vi "FGV Drift Daten.vi"(0 "SpanRegister":refnum<vi>, 1 "0-Gas Wert?":bool, 5 "Testnr.":i32, 7 "Drift Konfig Daten":T10={"Bearbeiter:"="", "Pfad:"=path "D:/IAG_Data/Log", "Textname:"="", "CG Aufschaltzeit:"=120.0, "N2 Aufschaltzeit:"=120.0} {"N2 Aufschaltzeit:" min=10.0; "CG Aufschaltzeit:" min=10.0}, 9 "Spangaseinstellungen":T2[](array[typedef]) {"Komponenten"."Komponente 5"."Komponente:" items=["NO (350,3000) LP 191C", "NO2 (150) LP 191C (1of2)", "NO2 (2000) LP 191C (2of2)", "N2O (300) LP 191C (1of2)", "NH3 (300) LP 191C (1of2)", "NH3 (900,3000) LP 191C (2of2)", "HNCO (400) 191C", "H2O% (30) LP 191C", "Formaldehyde (70,500) LP 191C", "CO2 low% (4) LP 191C (2of2)", "CO2% (20) LP 191C (1of2)", "CO (700) LP 191C (1of3)", "CO% (1) LP 191C (2of3)", "Propylene (1000) LP 191C", "Aromatic HC C7 (500) LP 191C", "Ethylene (1000) LP 191C", "CH4 (250) LP 191C (1of2)", "CH4 (5000) LP 191C (2of2)", "Ethane (1000) LP 191C", "Acetylene (1000) LP 191C", "HNO2 (20) 191C", "MeOH (1000) 191C", "CO% (10) LP 191C (3of3)", "Formic Acid (100) 191C", "SO2 (500) LP 191C", "Acetaldehyde (1000) LP 191C", "COS (100) LP 191C", "1,3 butadiene (100) LP 191C", "Oil as Octane (200) LP 191C", "N2O (1000) LP 191C (2of2)", "Propane (200) LP 191C", "NO2 autorange (2000)", "CO autorange (100000)", "CH4 autorange (5000)", "NH3 autorange (3000)", "Temp. Gascell", "Pressure Gascell", "sBeam@2500"]; "Komponenten"."Komponente 5"."Konzentration IST" format="%#.4f"; "Komponenten"."Komponente 5"."Genauigkeit" format="%#.1f"; "Komponenten"."Komponente 4"."Komponente:" items=["NO (350,3000) LP 191C", "NO2 (150) LP 191C (1of2)", "NO2 (2000) LP 191C (2of2)", "N2O (300) LP 191C (1of2)", "NH3 (300) LP 191C (1of2)", "NH3 (900,3000) LP 191C (2of2)", "HNCO (400) 191C", "H2O% (30) LP 191C", "Formaldehyde (70,500) LP 191C", "CO2 low% (4) LP 191C (2of2)", "CO2% (20) LP 191C (1of2)", "CO (700) LP 191C (1of3)", "CO% (1) LP 191C (2of3)", "Propylene (1000) LP 191C", "Aromatic HC C7 (500) LP 191C", "Ethylene (1000) LP 191C", "CH4 (250) LP 191C (1of2)", "CH4 (5000) LP 191C (2of2)", "Ethane (1000) LP 191C", "Acetylene (1000) LP 191C", "HNO2 (20) 191C", "MeOH (1000) 191C", "CO% (10) LP 191C (3of3)", "Formic Acid (100) 191C", "SO2 (500) LP 191C", "Acetaldehyde (1000) LP 191C", "COS (100) LP 191C", "1,3 butadiene (100) LP 191C", "Oil as Octane (200) LP 191C", "N2O (1000) LP 191C (2of2)", "Propane (200) LP 191C", "NO2 autorange (2000)", "CO autorange (100000)", "CH4 autorange (5000)", "NH3 autorange (3000)", "Temp. Gascell", "Pressure Gascell", "sBeam@2500"]; "Komponenten"."Komponente 4"."Konzentration IST" format="%#.4f"; "Komponenten"."Komponente 4"."Genauigkeit" format="%#.1f"; "Komponenten"."Komponente 3"."Komponente:" items=["NO (350,3000) LP 191C", "NO2 (150) LP 191C (1of2)", "NO2 (2000) LP 191C (2of2)", "N2O (300) LP 191C (1of2)", "NH3 (300) LP 191C (1of2)", "NH3 (900,3000) LP 191C (2of2)", "HNCO (400) 191C", "H2O% (30) LP 191C", "Formaldehyde (70,500) LP 191C", "CO2 low% (4) LP 191C (2of2)", "CO2% (20) LP 191C (1of2)", "CO (700) LP 191C (1of3)", "CO% (1) LP 191C (2of3)", "Propylene (1000) LP 191C", "Aromatic HC C7 (500) LP 191C", "Ethylene (1000) LP 191C", "CH4 (250) LP 191C (1of2)", "CH4 (5000) LP 191C (2of2)", "Ethane (1000) LP 191C", "Acetylene (1000) LP 191C", "HNO2 (20) 191C", "MeOH (1000) 191C", "CO% (10) LP 191C (3of3)", "Formic Acid (100) 191C", "SO2 (500) LP 191C", "Acetaldehyde (1000) LP 191C", "COS (100) LP 191C", "1,3 butadiene (100) LP 191C", "Oil as Octane (200) LP 191C", "N2O (1000) LP 191C (2of2)", "Propane (200) LP 191C", "NO2 autorange (2000)", "CO autorange (100000)", "CH4 autorange (5000)", "NH3 autorange (3000)", "Temp. Gascell", "Pressure Gascell", "sBeam@2500"]; "Komponenten"."Komponente 3"."Konzentration IST" format="%#.4f"; "Komponenten"."Komponente 3"."Genauigkeit" format="%#.1f"; "Komponenten"."Komponente 2"."Komponente:" items=["NO (350,3000) LP 191C", "NO2 (150) LP 191C (1of2)", "NO2 (2000) LP 191C (2of2)", "N2O (300) LP 191C (1of2)", "NH3 (300) LP 191C (1of2)", "NH3 (900,3000) LP 191C (2of2)", "HNCO (400) 191C", "H2O% (30) LP 191C", "Formaldehyde (70,500) LP 191C", "CO2 low% (4) LP 191C (2of2)", "CO2% (20) LP 191C (1of2)", "CO (700) LP 191C (1of3)", "CO% (1) LP 191C (2of3)", "Propylene (1000) LP 191C", "Aromatic HC C7 (500) LP 191C", "Ethylene (1000) LP 191C", "CH4 (250) LP 191C (1of2)", "CH4 (5000) LP 191C (2of2)", "Ethane (1000) LP 191C", "Acetylene (1000) LP 191C", "HNO2 (20) 191C", "MeOH (1000) 191C", "CO% (10) LP 191C (3of3)", "Formic Acid (100) 191C", "SO2 (500) LP 191C", "Acetaldehyde (1000) LP 191C", "COS (100) LP 191C", "1,3 butadiene (100) LP 191C", "Oil as Octane (200) LP 191C", "N2O (1000) LP 191C (2of2)", "Propane (200) LP 191C", "NO2 autorange (2000)", "CO autorange (100000)", "CH4 autorange (5000)", "NH3 autorange (3000)", "Temp. Gascell", "Pressure Gascell", "sBeam@2500"]; "Komponenten"."Komponente 2"."Konzentration IST" format="%#.4f"; "Komponenten"."Komponente 2"."Genauigkeit" format="%#.1f"; "Komponenten"."Komponente 1"."Komponente:" items=["NO (350,3000) LP 191C", "NO2 (150) LP 191C (1of2)", "NO2 (2000) LP 191C (2of2)", "N2O (300) LP 191C (1of2)", "NH3 (300) LP 191C (1of2)", "NH3 (900,3000) LP 191C (2of2)", "HNCO (400) 191C", "H2O% (30) LP 191C", "Formaldehyde (70,500) LP 191C", "CO2 low% (4) LP 191C (2of2)", "CO2% (20) LP 191C (1of2)", "CO (700) LP 191C (1of3)", "CO% (1) LP 191C (2of3)", "Propylene (1000) LP 191C", "Aromatic HC C7 (500) LP 191C", "Ethylene (1000) LP 191C", "CH4 (250) LP 191C (1of2)", "CH4 (5000) LP 191C (2of2)", "Ethane (1000) LP 191C", "Acetylene (1000) LP 191C", "HNO2 (20) 191C", "MeOH (1000) 191C", "CO% (10) LP 191C (3of3)", "Formic Acid (100) 191C", "SO2 (500) LP 191C", "Acetaldehyde (1000) LP 191C", "COS (100) LP 191C", "1,3 butadiene (100) LP 191C", "Oil as Octane (200) LP 191C", "N2O (1000) LP 191C (2of2)", "Propane (200) LP 191C", "NO2 autorange (2000)", "CO autorange (100000)", "CH4 autorange (5000)", "NH3 autorange (3000)", "Temp. Gascell", "Pressure Gascell", "sBeam@2500"]; "Komponenten"."Komponente 1"."Konzentration IST" format="%#.4f"; "Komponenten"."Komponente 1"."Genauigkeit" format="%#.1f"; "Modus" items=["Cal Gas to PNS", "Cal Gas to Samplepoint"]; "Ablaufdatum" format="%<%d.%m.%Y>T"; "Gasflasche" items=["----"=10000, "IAG NH3 3000"=0, "IAG NH3 200"=1, "IAG NH3 2000"=2, "IAG MG"=3, "IAG O2"=4]}, 11 "error in (no error)":errorcluster caption="Fehler (Eingang, kein Fehler)", 12 "Fehlercluster":T1(array[cluster]), 13 "Aktion":T11) -> (2 "PDF Pfad":path, 3 "Tabellenbeginn":i32[](array[numeric]), 4 "Drifttabelle":T9, 6 "keine Pre Daten vorhanden":bool, 8 "Drift Konfig Daten":T10={"Bearbeiter:"="", "Pfad:"=path "D:/IAG_Data/Log", "Textname:"="", "CG Aufschaltzeit:"=120.0, "N2 Aufschaltzeit:"=120.0} {"N2 Aufschaltzeit:" min=10.0; "CG Aufschaltzeit:" min=10.0}, 10 "Spangaseinstellungen":T2[](array[typedef]) {"Komponenten"."Komponente 5"."Komponente:" items=["NO (350,3000) LP 191C", "NO2 (150) LP 191C (1of2)", "NO2 (2000) LP 191C (2of2)", "N2O (300) LP 191C (1of2)", "NH3 (300) LP 191C (1of2)", "NH3 (900,3000) LP 191C (2of2)", "HNCO (400) 191C", "H2O% (30) LP 191C", "Formaldehyde (70,500) LP 191C", "CO2 low% (4) LP 191C (2of2)", "CO2% (20) LP 191C (1of2)", "CO (700) LP 191C (1of3)", "CO% (1) LP 191C (2of3)", "Propylene (1000) LP 191C", "Aromatic HC C7 (500) LP 191C", "Ethylene (1000) LP 191C", "CH4 (250) LP 191C (1of2)", "CH4 (5000) LP 191C (2of2)", "Ethane (1000) LP 191C", "Acetylene (1000) LP 191C", "HNO2 (20) 191C", "MeOH (1000) 191C", "CO% (10) LP 191C (3of3)", "Formic Acid (100) 191C", "SO2 (500) LP 191C", "Acetaldehyde (1000) LP 191C", "COS (100) LP 191C", "1,3 butadiene (100) LP 191C", "Oil as Octane (200) LP 191C", "N2O (1000) LP 191C (2of2)", "Propane (200) LP 191C", "NO2 autorange (2000)", "CO autorange (100000)", "CH4 autorange (5000)", "NH3 autorange (3000)", "Temp. Gascell", "Pressure Gascell", "sBeam@2500"]; "Komponenten"."Komponente 5"."Konzentration IST" format="%#.4f"; "Komponenten"."Komponente 5"."Genauigkeit" format="%#.1f"; "Komponenten"."Komponente 4"."Komponente:" items=["NO (350,3000) LP 191C", "NO2 (150) LP 191C (1of2)", "NO2 (2000) LP 191C (2of2)", "N2O (300) LP 191C (1of2)", "NH3 (300) LP 191C (1of2)", "NH3 (900,3000) LP 191C (2of2)", "HNCO (400) 191C", "H2O% (30) LP 191C", "Formaldehyde (70,500) LP 191C", "CO2 low% (4) LP 191C (2of2)", "CO2% (20) LP 191C (1of2)", "CO (700) LP 191C (1of3)", "CO% (1) LP 191C (2of3)", "Propylene (1000) LP 191C", "Aromatic HC C7 (500) LP 191C", "Ethylene (1000) LP 191C", "CH4 (250) LP 191C (1of2)", "CH4 (5000) LP 191C (2of2)", "Ethane (1000) LP 191C", "Acetylene (1000) LP 191C", "HNO2 (20) 191C", "MeOH (1000) 191C", "CO% (10) LP 191C (3of3)", "Formic Acid (100) 191C", "SO2 (500) LP 191C", "Acetaldehyde (1000) LP 191C", "COS (100) LP 191C", "1,3 butadiene (100) LP 191C", "Oil as Octane (200) LP 191C", "N2O (1000) LP 191C (2of2)", "Propane (200) LP 191C", "NO2 autorange (2000)", "CO autorange (100000)", "CH4 autorange (5000)", "NH3 autorange (3000)", "Temp. Gascell", "Pressure Gascell", "sBeam@2500"]; "Komponenten"."Komponente 4"."Konzentration IST" format="%#.4f"; "Komponenten"."Komponente 4"."Genauigkeit" format="%#.1f"; "Komponenten"."Komponente 3"."Komponente:" items=["NO (350,3000) LP 191C", "NO2 (150) LP 191C (1of2)", "NO2 (2000) LP 191C (2of2)", "N2O (300) LP 191C (1of2)", "NH3 (300) LP 191C (1of2)", "NH3 (900,3000) LP 191C (2of2)", "HNCO (400) 191C", "H2O% (30) LP 191C", "Formaldehyde (70,500) LP 191C", "CO2 low% (4) LP 191C (2of2)", "CO2% (20) LP 191C (1of2)", "CO (700) LP 191C (1of3)", "CO% (1) LP 191C (2of3)", "Propylene (1000) LP 191C", "Aromatic HC C7 (500) LP 191C", "Ethylene (1000) LP 191C", "CH4 (250) LP 191C (1of2)", "CH4 (5000) LP 191C (2of2)", "Ethane (1000) LP 191C", "Acetylene (1000) LP 191C", "HNO2 (20) 191C", "MeOH (1000) 191C", "CO% (10) LP 191C (3of3)", "Formic Acid (100) 191C", "SO2 (500) LP 191C", "Acetaldehyde (1000) LP 191C", "COS (100) LP 191C", "1,3 butadiene (100) LP 191C", "Oil as Octane (200) LP 191C", "N2O (1000) LP 191C (2of2)", "Propane (200) LP 191C", "NO2 autorange (2000)", "CO autorange (100000)", "CH4 autorange (5000)", "NH3 autorange (3000)", "Temp. Gascell", "Pressure Gascell", "sBeam@2500"]; "Komponenten"."Komponente 3"."Konzentration IST" format="%#.4f"; "Komponenten"."Komponente 3"."Genauigkeit" format="%#.1f"; "Komponenten"."Komponente 2"."Komponente:" items=["NO (350,3000) LP 191C", "NO2 (150) LP 191C (1of2)", "NO2 (2000) LP 191C (2of2)", "N2O (300) LP 191C (1of2)", "NH3 (300) LP 191C (1of2)", "NH3 (900,3000) LP 191C (2of2)", "HNCO (400) 191C", "H2O% (30) LP 191C", "Formaldehyde (70,500) LP 191C", "CO2 low% (4) LP 191C (2of2)", "CO2% (20) LP 191C (1of2)", "CO (700) LP 191C (1of3)", "CO% (1) LP 191C (2of3)", "Propylene (1000) LP 191C", "Aromatic HC C7 (500) LP 191C", "Ethylene (1000) LP 191C", "CH4 (250) LP 191C (1of2)", "CH4 (5000) LP 191C (2of2)", "Ethane (1000) LP 191C", "Acetylene (1000) LP 191C", "HNO2 (20) 191C", "MeOH (1000) 191C", "CO% (10) LP 191C (3of3)", "Formic Acid (100) 191C", "SO2 (500) LP 191C", "Acetaldehyde (1000) LP 191C", "COS (100) LP 191C", "1,3 butadiene (100) LP 191C", "Oil as Octane (200) LP 191C", "N2O (1000) LP 191C (2of2)", "Propane (200) LP 191C", "NO2 autorange (2000)", "CO autorange (100000)", "CH4 autorange (5000)", "NH3 autorange (3000)", "Temp. Gascell", "Pressure Gascell", "sBeam@2500"]; "Komponenten"."Komponente 2"."Konzentration IST" format="%#.4f"; "Komponenten"."Komponente 2"."Genauigkeit" format="%#.1f"; "Komponenten"."Komponente 1"."Komponente:" items=["NO (350,3000) LP 191C", "NO2 (150) LP 191C (1of2)", "NO2 (2000) LP 191C (2of2)", "N2O (300) LP 191C (1of2)", "NH3 (300) LP 191C (1of2)", "NH3 (900,3000) LP 191C (2of2)", "HNCO (400) 191C", "H2O% (30) LP 191C", "Formaldehyde (70,500) LP 191C", "CO2 low% (4) LP 191C (2of2)", "CO2% (20) LP 191C (1of2)", "CO (700) LP 191C (1of3)", "CO% (1) LP 191C (2of3)", "Propylene (1000) LP 191C", "Aromatic HC C7 (500) LP 191C", "Ethylene (1000) LP 191C", "CH4 (250) LP 191C (1of2)", "CH4 (5000) LP 191C (2of2)", "Ethane (1000) LP 191C", "Acetylene (1000) LP 191C", "HNO2 (20) 191C", "MeOH (1000) 191C", "CO% (10) LP 191C (3of3)", "Formic Acid (100) 191C", "SO2 (500) LP 191C", "Acetaldehyde (1000) LP 191C", "COS (100) LP 191C", "1,3 butadiene (100) LP 191C", "Oil as Octane (200) LP 191C", "N2O (1000) LP 191C (2of2)", "Propane (200) LP 191C", "NO2 autorange (2000)", "CO autorange (100000)", "CH4 autorange (5000)", "NH3 autorange (3000)", "Temp. Gascell", "Pressure Gascell", "sBeam@2500"]; "Komponenten"."Komponente 1"."Konzentration IST" format="%#.4f"; "Komponenten"."Komponente 1"."Genauigkeit" format="%#.1f"; "Modus" items=["Cal Gas to PNS", "Cal Gas to Samplepoint"]; "Ablaufdatum" format="%<%d.%m.%Y>T"; "Gasflasche" items=["----"=10000, "IAG NH3 3000"=0, "IAG NH3 200"=1, "IAG NH3 2000"=2, "IAG MG"=3, "IAG O2"=4]}, 14 "Verwendete Spangaseingänge":i32[](array[numeric]), 15 "error out":errorcluster caption="Fehler (Ausgang)")   [LabVIEW 2020, in "EPA 1065.lvlib" / "Gas Analyzer Drift 1065-550.lvlib"]
uses:
  Gas Analyzer Drift 1065-550.lvlib
  Konfig Daten Drift Verification.ctl
  Chiller NO2 1065-376/Aktion FGV Drift Daten.ctl
  Drifttabelle.ctl
  Spaninlet Cluster.ctl
  Seiten/System Einstellungen V2/Konfig Gasflasche.ctl
  Seiten/System Einstellungen V2/Analysatoren.ctl
  Seiten/System Einstellungen V2/Gasflasche Auswahl.ctl
  T90 1065-308/Modus.ctl
  Komponentencluster.ctl
  Komponentenauswahl.ctl
  Linearisierung V2/Protokoll/Protokoll.lvlib
  Allgemein/allgemeine Sub-VIs.lvlib
  Seiten/System Einstellungen V2/System Einstellungen V2.lvlib
  T90 1065-308/T90 Test 1065-308.lvlib
panel:
  out "Zahl":u32
  # "Komponente"
  # "Konzentration"
  # "Einheit"
  # "Genauigkeit [%]"
  # "Komponente"
  # "Konzentration"
  # "Einheit"
  # "Genauigkeit [%]"
  # "sec."
  # "sec."
  # "sec."
  # "sec."
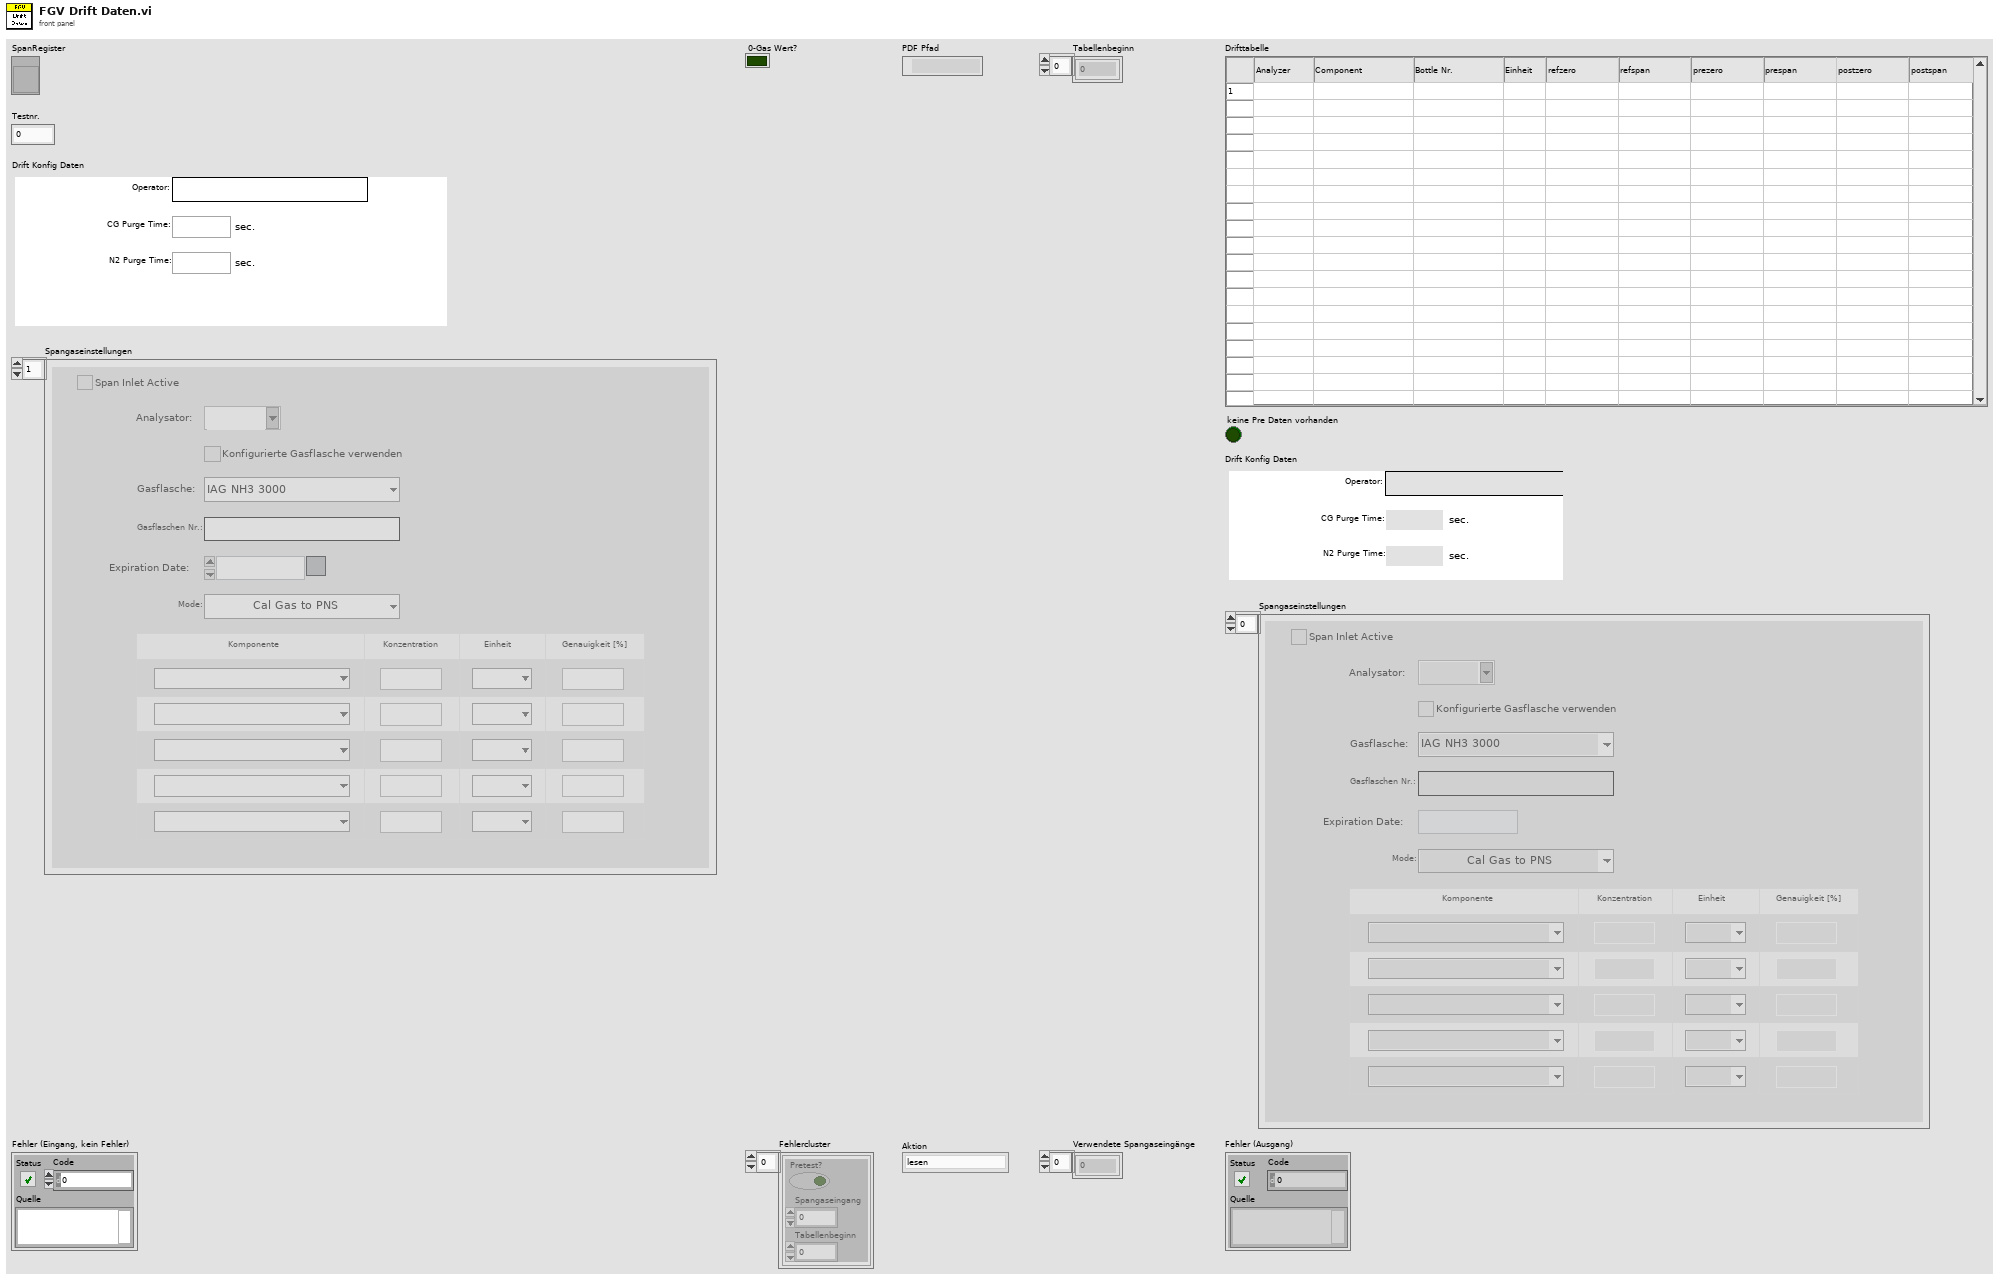
[diagram p1: front panel]
types:
  T1 = cluster{"Pretest?":bool, "Spangaseingang":i32, "Tabellenbeginn":i32}[]
  T2 = typedef "EPA 1065.lvlib/Gas Analyzer Drift 1065-550.lvlib/Spaninlet Cluster.ctl" = cluster{"Span Inlet Active":T3, "Analysator":T4, "Konfig Gasflasche":T3, "Gasflasche":T5, "Gasflaschen Nr.:":string, "Ablaufdatum":timestamp, "Modus":T6, "Komponenten":T7}
  T3 = typedef "System Einstellungen V2.lvlib/Konfig Gasflasche.ctl" = bool
  T4 = typedef "System Einstellungen V2.lvlib/Analysatoren.ctl" = string
  T5 = typedef "System Einstellungen V2.lvlib/Gasflasche Auswahl.ctl" = u16
  T6 = typedef "EPA 1065.lvlib/T90 Test 1065-308.lvlib/Modus.ctl" = u16
  T7 = typedef "EPA 1065.lvlib/Gas Analyzer Drift 1065-550.lvlib/Komponentencluster.ctl" = cluster{"Komponente 1":T8, "Komponente 2":T8, "Komponente 3":T8, "Komponente 4":T8, "Komponente 5":T8}
  T8 = typedef "EPA 1065.lvlib/Gas Analyzer Drift 1065-550.lvlib/Komponentenauswahl.ctl" = cluster{"Komponente:":u16, "Konzentration IST":dbl, "Einheit":enum16{"ppm", "%"}, "Genauigkeit":dbl}
  T9 = typedef "EPA 1065.lvlib/Gas Analyzer Drift 1065-550.lvlib/Drifttabelle.ctl" = string[][]
  T10 = typedef "EPA 1065.lvlib/Gas Analyzer Drift 1065-550.lvlib/Konfig Daten Drift Verification.ctl" = cluster{"Bearbeiter:":string, "Pfad:":path, "Textname:":string, "CG Aufschaltzeit:":dbl, "N2 Aufschaltzeit:":dbl}
  T11 = typedef "EPA 1065.lvlib/Gas Analyzer Drift 1065-550.lvlib/Aktion FGV Drift Daten.ctl" = enum16{"lesen", "Konfig Daten", "PDF einstellen", "laden", "speichern", "Tabelle init", "Zeile Prüfen", "Info schreiben", "Span Einstellung", "Pre Werte schreiben", "Post Werte schreiben", "NB Pre Wert schreiben", "NB Post Wert schreiben", "Tabelle löschen"}
  T12 = enum16{"open", "replace", "create", "open or create", "replace or create", "replace or create with confirmation"}
  T13 = cluster{"Drift Konfig Daten":T10, "Spangaseinstellungen":T2[]}
  T14 = typedef "String - Ausgabefeld.ctl" = string
  T15 = cluster{"Pretest?":bool, "Spangaseingang":i32, "Tabellenbeginn":i32}
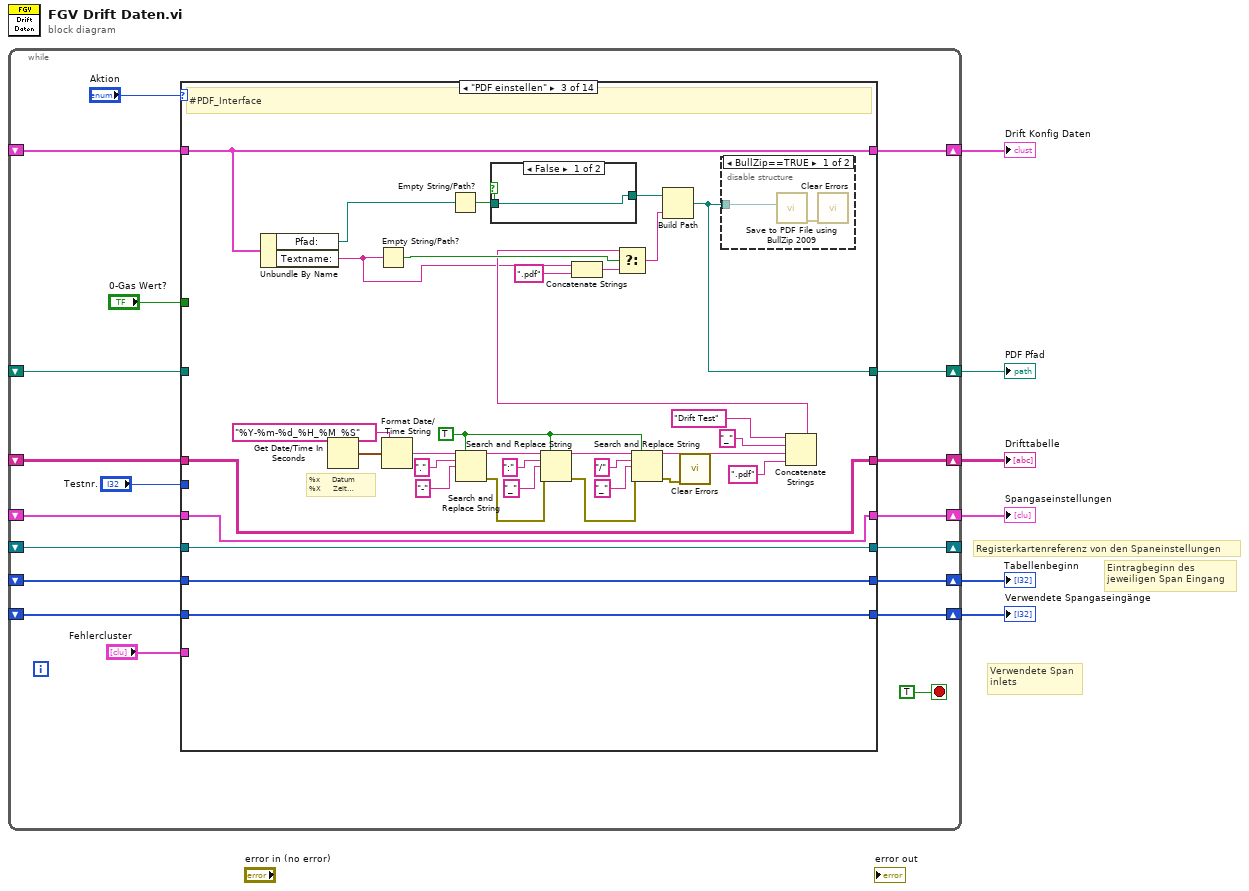
[diagram p0: block diagram]
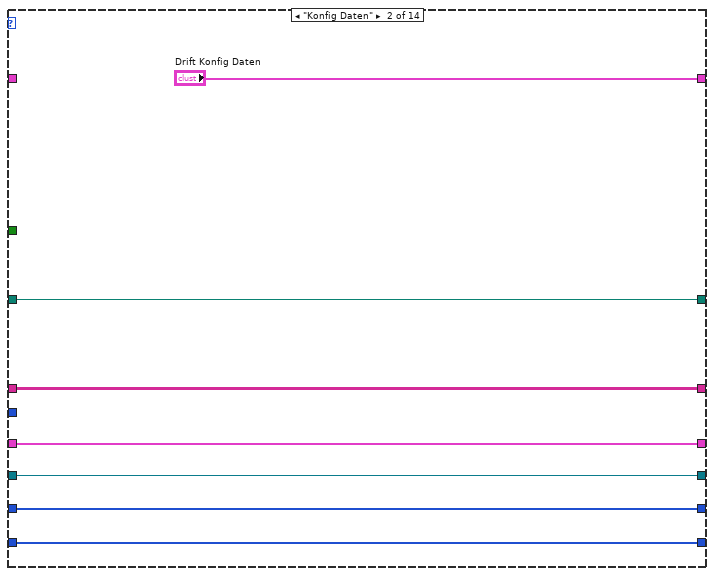
[diagram p3: hidden frame]
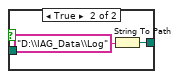
[diagram p5: hidden frame]
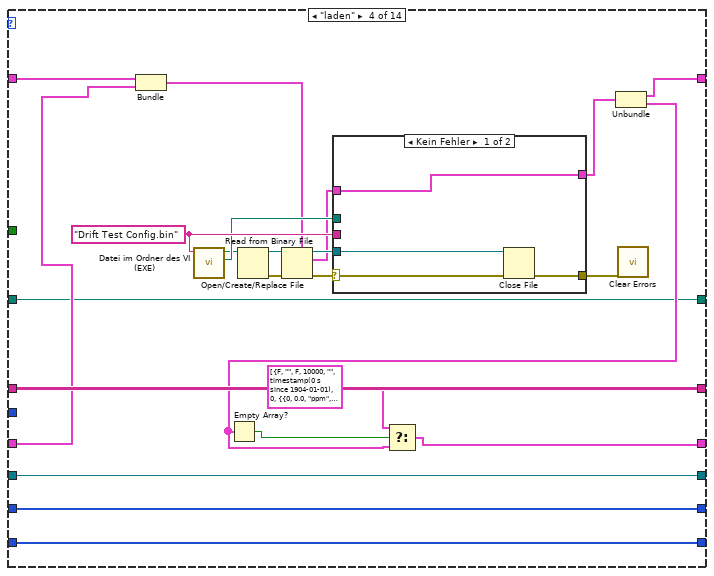
[diagram p6: hidden frame]
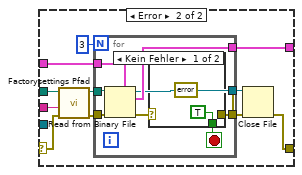
[diagram p7: hidden frame]
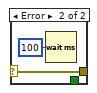
[diagram p8: hidden frame]
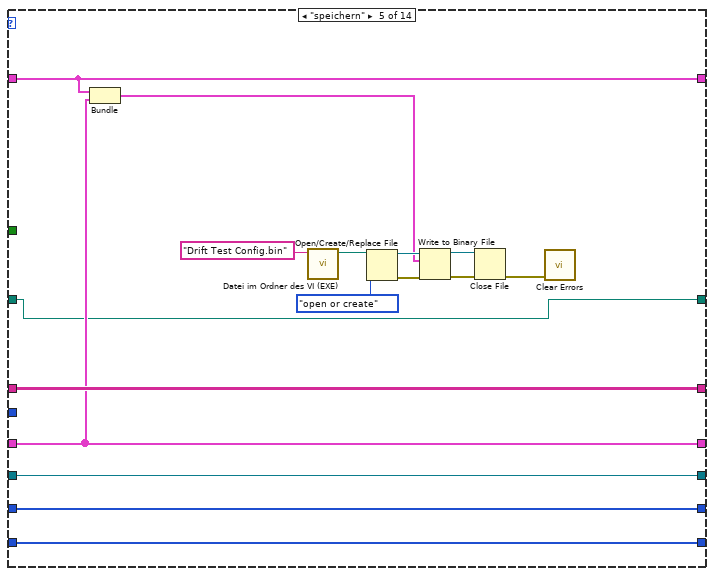
[diagram p9: hidden frame]
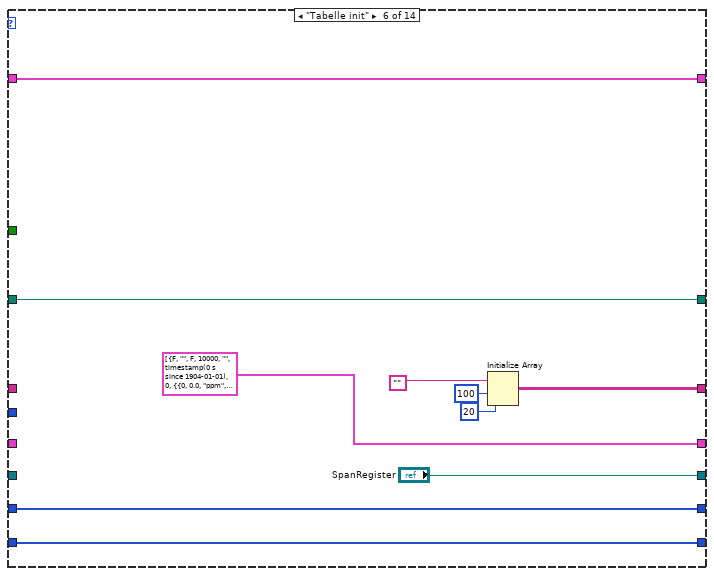
[diagram p10: hidden frame]
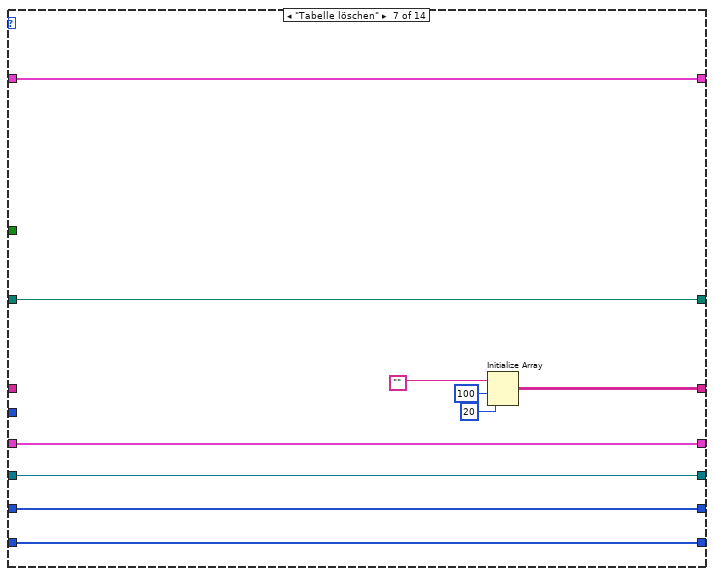
[diagram p11: hidden frame]
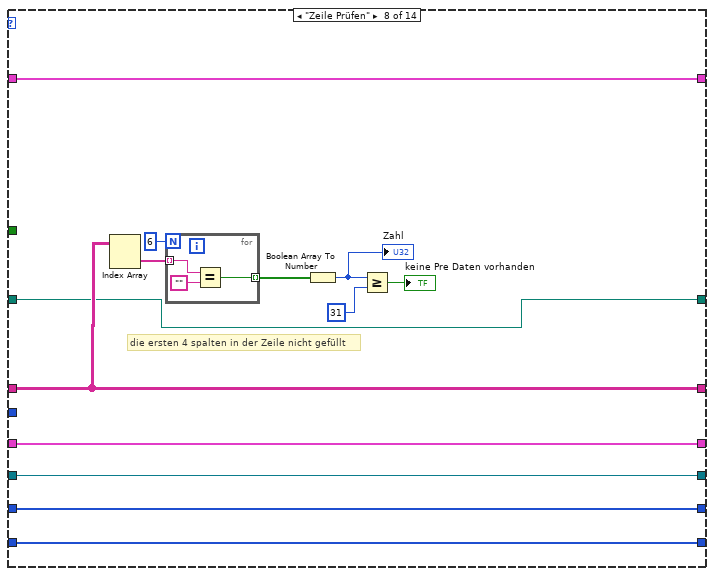
[diagram p12: hidden frame]
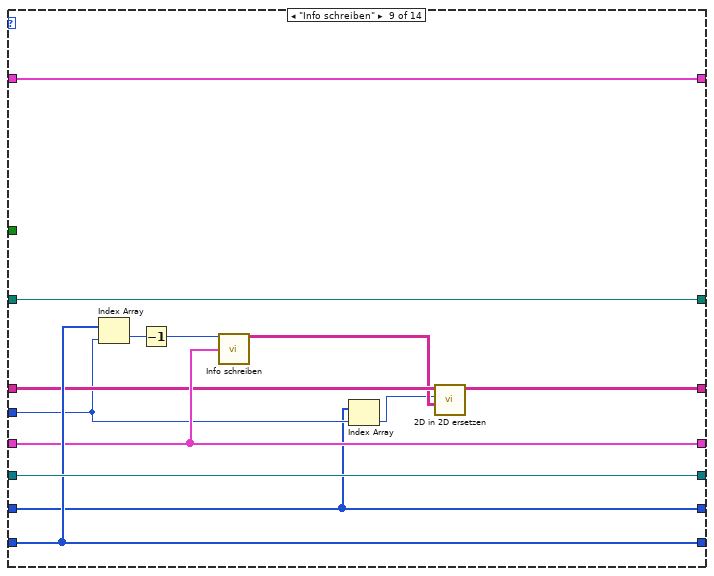
[diagram p13: hidden frame]
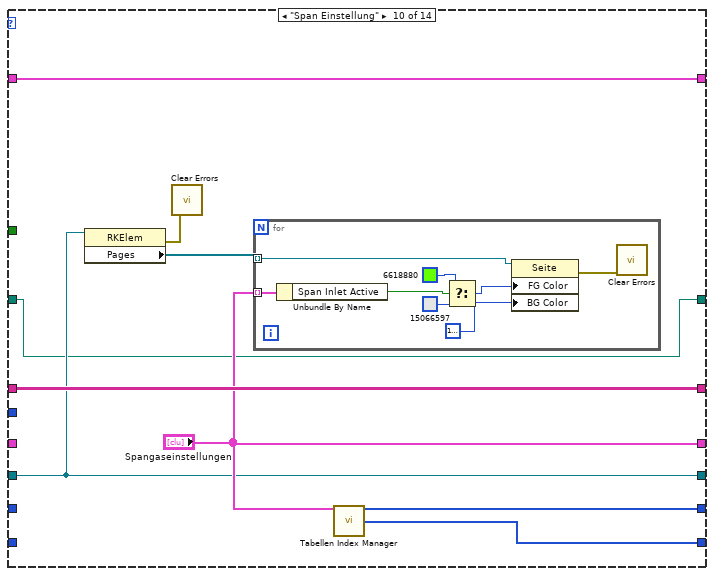
[diagram p14: hidden frame]
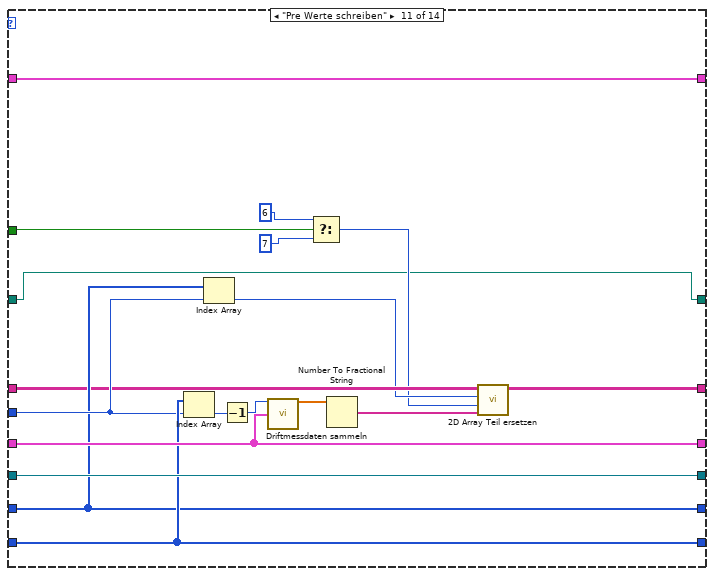
[diagram p15: hidden frame]
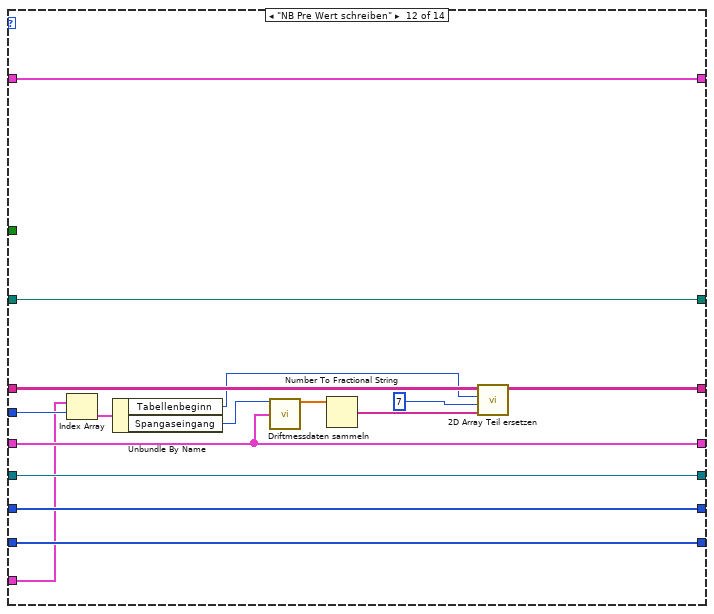
[diagram p16: hidden frame]
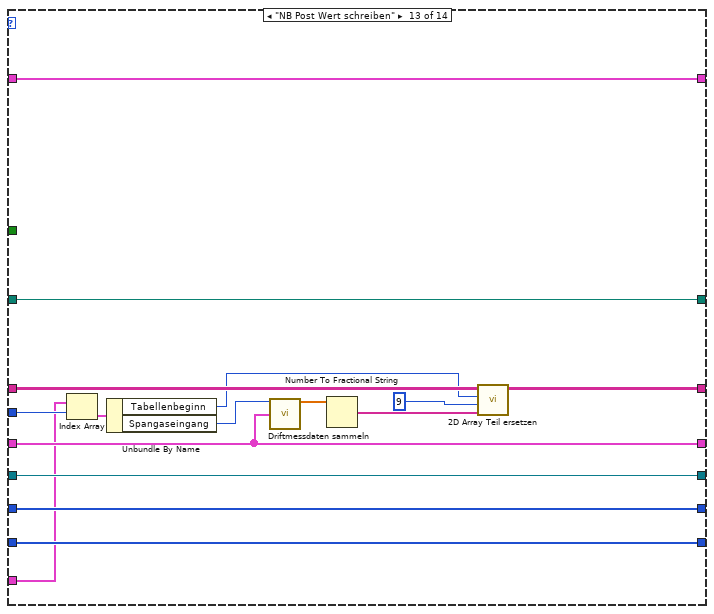
[diagram p17: hidden frame]
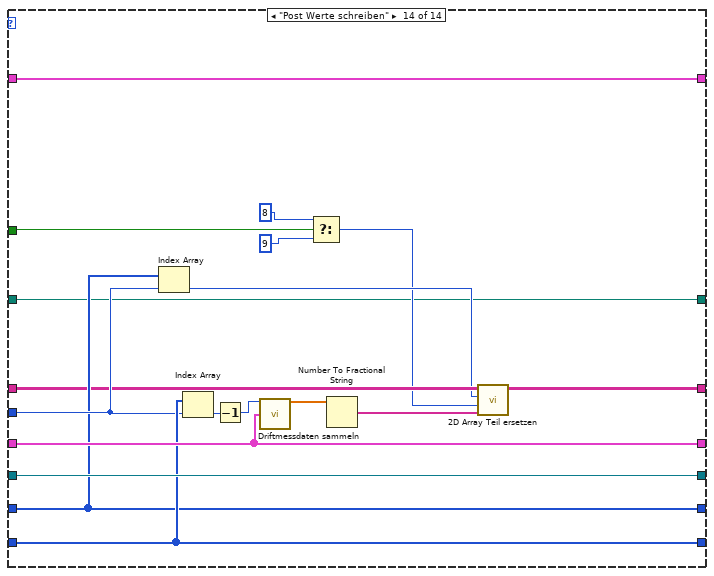
[diagram p18: hidden frame]
diagram:
  # "Registerkartenreferenz von den Spaneinstellungen"
  # "Eintragbeginn des\njeweiligen Span Eingang"
  # "Verwendete Span\ninlets"
  n1 = while {
    shift-right: [w23] -> w6
    shift-left: _ -> [w20]
    shift-right: [w22] -> w5
    shift-left: _ -> [w21]
    shift-right: [w19] -> w4
    shift-left: _ -> [w18]
    shift-right: [w17] -> _
    shift-left: _ -> [w16]
    shift-right: [w15] -> w2
    shift-left: _ -> [w14]
    shift-right: [w12] -> w3
    shift-left: _ -> [w11]
    shift-right: [w8] -> w1
    shift-left: _ -> [w7]
    stop <- TRUE stop-if-true
    n2 = case shown="\"PDF einstellen\"" "Aktion" {
      tunnel: [w32 "Drift Konfig Daten" w74 w88 w135 w155 w165 w178 w194 w203 w228 w244 w260 w278] -> w23
      tunnel: w20 -> [w32 _ w74 w91 w135 w155 w165 w178 w194 w203 w228 w244 w260 w278]
      tunnel: [w31 w38 w48 w93 w138 w153 w163 w176 w188 w202 w220 w238 w254 w271] -> w22
      tunnel: w21 -> [w31 w38 w48 w93 w138 _ _ w176 w189 w202 w221 w239 w255 w272]
      tunnel: [w30 w37 w44 w81 w134 T2[] [{"Span Inlet Active"=FALSE, "Analysator"="", "Konfig Gasflasche"=FALSE, "Gasflasche"=10000, "Gasflaschen Nr.:"="", "Ablaufdatum"=timestamp(0 s since 1904-01-01), "Modus"=0, "Komponenten"={"Komponente 1"={"Komponente:"=0, "Konzentration IST"=0.0, "Einheit"=enum."ppm", "Genauigkeit"=0.0}, "Komponente 2"={"Komponente:"=0, "Konzentration IST"=0.0, "Einheit"=enum."ppm", "Genauigkeit"=0.0}, "Komponente 3"={"Komponente:"=0, "Konzentration IST"=0.0, "Einheit"=enum."ppm", "Genauigkeit"=0.0}, "Komponente 4"={"Komponente:"=0, "Konzentration IST"=0.0, "Einheit"=enum."ppm", "Genauigkeit"=0.0}, "Komponente 5"={"Komponente:"=0, "Konzentration IST"=0.0, "Einheit"=enum."ppm", "Genauigkeit"=0.0}}}, {"Span Inlet Active"=FALSE, "Analysator"="", "Konfig Gasflasche"=FALSE, "Gasflasche"=10000, "Gasflaschen Nr.:"="", "Ablaufdatum"=timestamp(0 s since 1904-01-01), "Modus"=0, "Komponenten"={"Komponente 1"={"Komponente:"=0, "Konzentration IST"=0.0, "Einheit"=enum."ppm", "Genauigkeit"=0.0}, "Komponente 2"={"Komponente:"=0, "Konzentration IST"=0.0, "Einheit"=enum."ppm", "Genauigkeit"=0.0}, "Komponente 3"={"Komponente:"=0, "Konzentration IST"=0.0, "Einheit"=enum."ppm", "Genauigkeit"=0.0}, "Komponente 4"={"Komponente:"=0, "Konzentration IST"=0.0, "Einheit"=enum."ppm", "Genauigkeit"=0.0}, "Komponente 5"={"Komponente:"=0, "Konzentration IST"=0.0, "Einheit"=enum."ppm", "Genauigkeit"=0.0}}}, {"Span Inlet Active"=FALSE, "Analysator"="", "Konfig Gasflasche"=FALSE, "Gasflasche"=10000, "Gasflaschen Nr.:"="", "Ablaufdatum"=timestamp(0 s since 1904-01-01), "Modus"=0, "Komponenten"={"Komponente 1"={"Komponente:"=0, "Konzentration IST"=0.0, "Einheit"=enum."ppm", "Genauigkeit"=0.0}, "Komponente 2"={"Komponente:"=0, "Konzentration IST"=0.0, "Einheit"=enum."ppm", "Genauigkeit"=0.0}, "Komponente 3"={"Komponente:"=0, "Konzentration IST"=0.0, "Einheit"=enum."ppm", "Genauigkeit"=0.0}, "Komponente 4"={"Komponente:"=0, "Konzentration IST"=0.0, "Einheit"=enum."ppm", "Genauigkeit"=0.0}, "Komponente 5"={"Komponente:"=0, "Konzentration IST"=0.0, "Einheit"=enum."ppm", "Genauigkeit"=0.0}}}, {"Span Inlet Active"=FALSE, "Analysator"="", "Konfig Gasflasche"=FALSE, "Gasflasche"=10000, "Gasflaschen Nr.:"="", "Ablaufdatum"=timestamp(0 s since 1904-01-01), "Modus"=0, "Komponenten"={"Komponente 1"={"Komponente:"=0, "Konzentration IST"=0.0, "Einheit"=enum."ppm", "Genauigkeit"=0.0}, "Komponente 2"={"Komponente:"=0, "Konzentration IST"=0.0, "Einheit"=enum."ppm", "Genauigkeit"=0.0}, "Komponente 3"={"Komponente:"=0, "Konzentration IST"=0.0, "Einheit"=enum."ppm", "Genauigkeit"=0.0}, "Komponente 4"={"Komponente:"=0, "Konzentration IST"=0.0, "Einheit"=enum."ppm", "Genauigkeit"=0.0}, "Komponente 5"={"Komponente:"=0, "Konzentration IST"=0.0, "Einheit"=enum."ppm", "Genauigkeit"=0.0}}}, {"Span Inlet Active"=FALSE, "Analysator"="", "Konfig Gasflasche"=FALSE, "Gasflasche"=10000, "Gasflaschen Nr.:"="", "Ablaufdatum"=timestamp(0 s since 1904-01-01), "Modus"=0, "Komponenten"={"Komponente 1"={"Komponente:"=0, "Konzentration IST"=0.0, "Einheit"=enum."ppm", "Genauigkeit"=0.0}, "Komponente 2"={"Komponente:"=0, "Konzentration IST"=0.0, "Einheit"=enum."ppm", "Genauigkeit"=0.0}, "Komponente 3"={"Komponente:"=0, "Konzentration IST"=0.0, "Einheit"=enum."ppm", "Genauigkeit"=0.0}, "Komponente 4"={"Komponente:"=0, "Konzentration IST"=0.0, "Einheit"=enum."ppm", "Genauigkeit"=0.0}, "Komponente 5"={"Komponente:"=0, "Konzentration IST"=0.0, "Einheit"=enum."ppm", "Genauigkeit"=0.0}}}, {"Span Inlet Active"=FALSE, "Analysator"="", "Konfig Gasflasche"=FALSE, "Gasflasche"=10000, "Gasflaschen Nr.:"="", "Ablaufdatum"=timestamp(0 s since 1904-01-01), "Modus"=0, "Komponenten"={"Komponente 1"={"Komponente:"=0, "Konzentration IST"=0.0, "Einheit"=enum."ppm", "Genauigkeit"=0.0}, "Komponente 2"={"Komponente:"=0, "Konzentration IST"=0.0, "Einheit"=enum."ppm", "Genauigkeit"=0.0}, "Komponente 3"={"Komponente:"=0, "Konzentration IST"=0.0, "Einheit"=enum."ppm", "Genauigkeit"=0.0}, "Komponente 4"={"Komponente:"=0, "Konzentration IST"=0.0, "Einheit"=enum."ppm", "Genauigkeit"=0.0}, "Komponente 5"={"Komponente:"=0, "Konzentration IST"=0.0, "Einheit"=enum."ppm", "Genauigkeit"=0.0}}}, {"Span Inlet Active"=FALSE, "Analysator"="", "Konfig Gasflasche"=FALSE, "Gasflasche"=10000, "Gasflaschen Nr.:"="", "Ablaufdatum"=timestamp(0 s since 1904-01-01), "Modus"=0, "Komponenten"={"Komponente 1"={"Komponente:"=0, "Konzentration IST"=0.0, "Einheit"=enum."ppm", "Genauigkeit"=0.0}, "Komponente 2"={"Komponente:"=0, "Konzentration IST"=0.0, "Einheit"=enum."ppm", "Genauigkeit"=0.0}, "Komponente 3"={"Komponente:"=0, "Konzentration IST"=0.0, "Einheit"=enum."ppm", "Genauigkeit"=0.0}, "Komponente 4"={"Komponente:"=0, "Konzentration IST"=0.0, "Einheit"=enum."ppm", "Genauigkeit"=0.0}, "Komponente 5"={"Komponente:"=0, "Konzentration IST"=0.0, "Einheit"=enum."ppm", "Genauigkeit"=0.0}}}, {"Span Inlet Active"=FALSE, "Analysator"="", "Konfig Gasflasche"=FALSE, "Gasflasche"=10000, "Gasflaschen Nr.:"="", "Ablaufdatum"=timestamp(0 s since 1904-01-01), "Modus"=0, "Komponenten"={"Komponente 1"={"Komponente:"=0, "Konzentration IST"=0.0, "Einheit"=enum."ppm", "Genauigkeit"=0.0}, "Komponente 2"={"Komponente:"=0, "Konzentration IST"=0.0, "Einheit"=enum."ppm", "Genauigkeit"=0.0}, "Komponente 3"={"Komponente:"=0, "Konzentration IST"=0.0, "Einheit"=enum."ppm", "Genauigkeit"=0.0}, "Komponente 4"={"Komponente:"=0, "Konzentration IST"=0.0, "Einheit"=enum."ppm", "Genauigkeit"=0.0}, "Komponente 5"={"Komponente:"=0, "Konzentration IST"=0.0, "Einheit"=enum."ppm", "Genauigkeit"=0.0}}}, {"Span Inlet Active"=FALSE, "Analysator"="", "Konfig Gasflasche"=FALSE, "Gasflasche"=10000, "Gasflaschen Nr.:"="", "Ablaufdatum"=timestamp(0 s since 1904-01-01), "Modus"=0, "Komponenten"={"Komponente 1"={"Komponente:"=0, "Konzentration IST"=0.0, "Einheit"=enum."ppm", "Genauigkeit"=0.0}, "Komponente 2"={"Komponente:"=0, "Konzentration IST"=0.0, "Einheit"=enum."ppm", "Genauigkeit"=0.0}, "Komponente 3"={"Komponente:"=0, "Konzentration IST"=0.0, "Einheit"=enum."ppm", "Genauigkeit"=0.0}, "Komponente 4"={"Komponente:"=0, "Konzentration IST"=0.0, "Einheit"=enum."ppm", "Genauigkeit"=0.0}, "Komponente 5"={"Komponente:"=0, "Konzentration IST"=0.0, "Einheit"=enum."ppm", "Genauigkeit"=0.0}}}, {"Span Inlet Active"=FALSE, "Analysator"="", "Konfig Gasflasche"=FALSE, "Gasflasche"=10000, "Gasflaschen Nr.:"="", "Ablaufdatum"=timestamp(0 s since 1904-01-01), "Modus"=0, "Komponenten"={"Komponente 1"={"Komponente:"=0, "Konzentration IST"=0.0, "Einheit"=enum."ppm", "Genauigkeit"=0.0}, "Komponente 2"={"Komponente:"=0, "Konzentration IST"=0.0, "Einheit"=enum."ppm", "Genauigkeit"=0.0}, "Komponente 3"={"Komponente:"=0, "Konzentration IST"=0.0, "Einheit"=enum."ppm", "Genauigkeit"=0.0}, "Komponente 4"={"Komponente:"=0, "Konzentration IST"=0.0, "Einheit"=enum."ppm", "Genauigkeit"=0.0}, "Komponente 5"={"Komponente:"=0, "Konzentration IST"=0.0, "Einheit"=enum."ppm", "Genauigkeit"=0.0}}}, {"Span Inlet Active"=FALSE, "Analysator"="", "Konfig Gasflasche"=FALSE, "Gasflasche"=10000, "Gasflaschen Nr.:"="", "Ablaufdatum"=timestamp(0 s since 1904-01-01), "Modus"=0, "Komponenten"={"Komponente 1"={"Komponente:"=0, "Konzentration IST"=0.0, "Einheit"=enum."ppm", "Genauigkeit"=0.0}, "Komponente 2"={"Komponente:"=0, "Konzentration IST"=0.0, "Einheit"=enum."ppm", "Genauigkeit"=0.0}, "Komponente 3"={"Komponente:"=0, "Konzentration IST"=0.0, "Einheit"=enum."ppm", "Genauigkeit"=0.0}, "Komponente 4"={"Komponente:"=0, "Konzentration IST"=0.0, "Einheit"=enum."ppm", "Genauigkeit"=0.0}, "Komponente 5"={"Komponente:"=0, "Konzentration IST"=0.0, "Einheit"=enum."ppm", "Genauigkeit"=0.0}}}] ("Spangaseinstellungen") w157 w170 w191 "Spangaseinstellungen" w226 w242 w258 w276] -> w19
      tunnel: w18 -> [w30 w37 w44 w87 w134 _ w157 w170 w191 _ w226 w242 w258 w276]
      tunnel: [w29 w36 w43 w92 w136 "SpanRegister" w158 w169 w193 w198 w227 w243 w259 w277] -> w17
      tunnel: w16 -> [w29 w36 w43 w92 w136 _ w158 w169 w193 w198 w227 w243 w259 w277]
      tunnel: [w28 w35 w42 w86 w132 w149 w160 w168 w185 w200 w222 w240 w256 w273] -> w15
      tunnel: w14 -> [w28 w35 w42 w86 w132 w149 w160 w168 w185 _ w222 w240 w256 w273]
      tunnel: "Testnr." -> [_ _ _ _ _ _ _ _ w186 _ w223 w235 w251 w274]
      tunnel: [w27 w34 w41 w85 w131 w148 w159 w167 w192 w199 w225 w241 w257 w275] -> w12
      tunnel: w11 -> [w27 w34 w41 w85 w131 w148 w159 w167 w192 _ w225 w241 w257 w275]
      tunnel: "0-Gas Wert?" -> [_ _ _ _ _ _ _ _ _ _ w217 _ _ w268]
      tunnel: "Fehlercluster" -> [_ _ _ _ _ _ _ _ _ _ _ w234 w250 _]
      tunnel: [w26 w33 w40 w80 w130 w146 w156 w166 w182 w195 w212 w230 w246 w262] -> w8
      tunnel: w7 -> [w26 w33 _ w80 w130 w146 w156 w166 w182 w195 w212 w230 w246 w262]
      frame "lesen", Default {
      }
      frame "Konfig Daten" {
      }
      frame "PDF einstellen" {
        w65 = TRUE ("Alle ersetzen? (F)")
        # "%x      Datum\n%X      Zeit (h:m:s)"
        # "#PDF_Interface"
        n3 = Unbundle By Name(w74) -> ("Pfad:"=w50:path, "Textname:"=w46:string)
        n4 = Get Date/Time In Seconds() -> (seconds since 1Jan1904=w73:timestamp)
        n5 = Empty String/Path?(string/path=w46) -> (empty?=w53:bool)
        n6 = Format Date/Time String(time format string (%c)="%Y-%m-%d_%H_%M_%S" ("Zeitformatierungs-String (%c)"), seconds (now)=w73) -> (date/time string=w72:string)  [unwired: 1 in]
        n7 = Empty String/Path?(string/path=w50) -> (empty?=w54:bool)
        n8 = Search and Replace String(replace all?=w65, input string=w72, search string="." ("Such-String"), replace string="-" ("String ersetzen(\"\")")) -> (result string=w71:string, error out=w68:errorcluster)  [unwired: 4 in, 2 out]
        n9 = case shown="False" w54 {
          tunnel: [w77 w78] -> w49
          tunnel: w50 -> [w77 _]
          frame False {
          }
          frame True {
            n10 = String To Path(string="D:\\IAG_Data\\Log" ("Pfad")) -> (path=w78:path)
          }
        }
        n11 = Search and Replace String(replace all?=w65, input string=w71, search string=":" ("Such-String"), replace string="_" ("String ersetzen(\"\")"), error in=w68) -> (result string=w70:string, error out=w67:errorcluster)  [unwired: 3 in, 2 out]
        n12 = Concatenate Strings(w46, ".pdf" ("String")) -> (w45:string)
        n13 = Search and Replace String(replace all?=w65, input string=w70, search string="/" ("Such-String"), replace string="_" ("String ersetzen(\"\")"), error in=w67) -> (result string=w69:string, error out=w66:errorcluster)  [unwired: 3 in, 2 out]
        n14 = call <vilib>:"Clear Errors.vi"("error in (no error)"=w66) -> ()  [unwired: 5 in, 2 out]
        n15 = Concatenate Strings("Drift Test" ("String"), "_", w69, ".pdf" ("String")) -> (w52:string)
        n16 = Select(t=w52, s=w53, f=w45) -> (s? t:f=w51:string)
        n17 = Build Path(base path=w49, name or relative path=w51) -> (appended path=w40:path)
        n18 = disable-structure shown="BullZip==TRUE" {
          disable-tunnel: w40 -> [w76 _]
          frame condition #0 {
            n19 = call "Save to PDF File using BullZip 2009.vi"("Save PDF File Path"=w76) -> ("error out"=w75:errorcluster)  [unwired: 10 in]
            n20 = call <vilib>:"Clear Errors.vi"("error in (no error)"=w75) -> ()  [unwired: 5 in, 2 out]
          }
          frame condition #1 (active) {
          }
        }
      }
      frame "laden" {
        w100 = "Drift Test Config.bin" ("Dateiname")
        n21 = Bundle("Drift Konfig Daten"=w91, "Spangaseinstellungen"=w87) -> (w90:T13)  [unwired: 1 in]
        n22 = call "Datei im Ordner des VI (EXE).vi"("Dateiname"=w100) -> ("Ordner des Haupt-VIs"=w99:path, "Dateipfad im Ordner des Haupt-VIs"=w96:path)  [unwired: 8 in, 1 out]
        n23 = Open/Create/Replace File(file path (use dialog)=w96) -> (refnum out=w94:refnum<file>, error out=w95:errorcluster)  [unwired: 5 in, 1 out]
        n24 = Read from Binary File(5:w90, 8:w95, 11:w94) -> (0:w102:errorcluster, 2:w97:T13, 3:w98:refnum<file>)  [unwired: 3 in, 1 out]
        n25 = case shown="Kein Fehler" w102 {
          selector: w102 -> [w105 w109]
          tunnel: w99 -> [_ w110]
          tunnel: w97 -> [w106 w108]
          tunnel: [w106 w116] -> w89
          tunnel: [w103 w114] -> w101
          tunnel: w98 -> [w104 _]
          tunnel: w100 -> [_ w107]
          frame No Error {
            n26 = Close File(refnum=w104, error in=w105) -> (error out=w103:errorcluster)  [unwired: 1 out]
          }
          frame Error {
            n27 = call "Factorysettings Pfad.vi"("error in (no error)"=w109, "Dateiname"=w107, "Ordner des Haupt-VIs"=w110) -> ("error out"=w111:errorcluster, "Pfad Factorysettings"=w112:path)  [unwired: 7 in]
            n28 = for {
              N: 3 -> [_]
              tunnel: w111 -> [w123]
              tunnel: w112 -> [w122]
              tunnel: [w121] -> w116
              tunnel: [w120] -> w115
              tunnel: [w119] -> w113
              tunnel: w108 -> [w118]
              stop <- w124 stop-if-true
              n29 = Read from Binary File(5:w118, 8:w123, 11:w122) -> (0:w125:errorcluster, 2:w121:T13, 3:w119:refnum<file>)  [unwired: 3 in, 1 out]
              n30 = case shown="Kein Fehler" w125 {
                selector: w125 -> [_ w128]
                tunnel: [TRUE _] -> w124
                tunnel: [errorcluster {"status"=FALSE, "code"=0, "source"=""} ("error IO") w128] -> w120
                frame No Error {
                }
                frame Error {
                  n31 = Wait (ms)(milliseconds to wait=u32 100 ("Zu wartende ms")) -> ()  [unwired: 1 out]
                }
              }
            }
            n32 = Close File(refnum=w113, error in=w115) -> (error out=w114:errorcluster)  [unwired: 1 out]
          }
        }
        n33 = Unbundle(w89) -> ("Drift Konfig Daten"=w88:T10, "Spangaseinstellungen"=w82:T2[])
        n34 = Empty Array?(array=w82) -> (empty?=w84:bool)
        n35 = Select(t=T2[] [{"Span Inlet Active"=FALSE, "Analysator"="", "Konfig Gasflasche"=FALSE, "Gasflasche"=10000, "Gasflaschen Nr.:"="", "Ablaufdatum"=timestamp(0 s since 1904-01-01), "Modus"=0, "Komponenten"={"Komponente 1"={"Komponente:"=0, "Konzentration IST"=0.0, "Einheit"=enum."ppm", "Genauigkeit"=0.0}, "Komponente 2"={"Komponente:"=0, "Konzentration IST"=0.0, "Einheit"=enum."ppm", "Genauigkeit"=0.0}, "Komponente 3"={"Komponente:"=0, "Konzentration IST"=0.0, "Einheit"=enum."ppm", "Genauigkeit"=0.0}, "Komponente 4"={"Komponente:"=0, "Konzentration IST"=0.0, "Einheit"=enum."ppm", "Genauigkeit"=0.0}, "Komponente 5"={"Komponente:"=0, "Konzentration IST"=0.0, "Einheit"=enum."ppm", "Genauigkeit"=0.0}}}, {"Span Inlet Active"=FALSE, "Analysator"="", "Konfig Gasflasche"=FALSE, "Gasflasche"=10000, "Gasflaschen Nr.:"="", "Ablaufdatum"=timestamp(0 s since 1904-01-01), "Modus"=0, "Komponenten"={"Komponente 1"={"Komponente:"=0, "Konzentration IST"=0.0, "Einheit"=enum."ppm", "Genauigkeit"=0.0}, "Komponente 2"={"Komponente:"=0, "Konzentration IST"=0.0, "Einheit"=enum."ppm", "Genauigkeit"=0.0}, "Komponente 3"={"Komponente:"=0, "Konzentration IST"=0.0, "Einheit"=enum."ppm", "Genauigkeit"=0.0}, "Komponente 4"={"Komponente:"=0, "Konzentration IST"=0.0, "Einheit"=enum."ppm", "Genauigkeit"=0.0}, "Komponente 5"={"Komponente:"=0, "Konzentration IST"=0.0, "Einheit"=enum."ppm", "Genauigkeit"=0.0}}}, {"Span Inlet Active"=FALSE, "Analysator"="", "Konfig Gasflasche"=FALSE, "Gasflasche"=10000, "Gasflaschen Nr.:"="", "Ablaufdatum"=timestamp(0 s since 1904-01-01), "Modus"=0, "Komponenten"={"Komponente 1"={"Komponente:"=0, "Konzentration IST"=0.0, "Einheit"=enum."ppm", "Genauigkeit"=0.0}, "Komponente 2"={"Komponente:"=0, "Konzentration IST"=0.0, "Einheit"=enum."ppm", "Genauigkeit"=0.0}, "Komponente 3"={"Komponente:"=0, "Konzentration IST"=0.0, "Einheit"=enum."ppm", "Genauigkeit"=0.0}, "Komponente 4"={"Komponente:"=0, "Konzentration IST"=0.0, "Einheit"=enum."ppm", "Genauigkeit"=0.0}, "Komponente 5"={"Komponente:"=0, "Konzentration IST"=0.0, "Einheit"=enum."ppm", "Genauigkeit"=0.0}}}, {"Span Inlet Active"=FALSE, "Analysator"="", "Konfig Gasflasche"=FALSE, "Gasflasche"=10000, "Gasflaschen Nr.:"="", "Ablaufdatum"=timestamp(0 s since 1904-01-01), "Modus"=0, "Komponenten"={"Komponente 1"={"Komponente:"=0, "Konzentration IST"=0.0, "Einheit"=enum."ppm", "Genauigkeit"=0.0}, "Komponente 2"={"Komponente:"=0, "Konzentration IST"=0.0, "Einheit"=enum."ppm", "Genauigkeit"=0.0}, "Komponente 3"={"Komponente:"=0, "Konzentration IST"=0.0, "Einheit"=enum."ppm", "Genauigkeit"=0.0}, "Komponente 4"={"Komponente:"=0, "Konzentration IST"=0.0, "Einheit"=enum."ppm", "Genauigkeit"=0.0}, "Komponente 5"={"Komponente:"=0, "Konzentration IST"=0.0, "Einheit"=enum."ppm", "Genauigkeit"=0.0}}}, {"Span Inlet Active"=FALSE, "Analysator"="", "Konfig Gasflasche"=FALSE, "Gasflasche"=10000, "Gasflaschen Nr.:"="", "Ablaufdatum"=timestamp(0 s since 1904-01-01), "Modus"=0, "Komponenten"={"Komponente 1"={"Komponente:"=0, "Konzentration IST"=0.0, "Einheit"=enum."ppm", "Genauigkeit"=0.0}, "Komponente 2"={"Komponente:"=0, "Konzentration IST"=0.0, "Einheit"=enum."ppm", "Genauigkeit"=0.0}, "Komponente 3"={"Komponente:"=0, "Konzentration IST"=0.0, "Einheit"=enum."ppm", "Genauigkeit"=0.0}, "Komponente 4"={"Komponente:"=0, "Konzentration IST"=0.0, "Einheit"=enum."ppm", "Genauigkeit"=0.0}, "Komponente 5"={"Komponente:"=0, "Konzentration IST"=0.0, "Einheit"=enum."ppm", "Genauigkeit"=0.0}}}, {"Span Inlet Active"=FALSE, "Analysator"="", "Konfig Gasflasche"=FALSE, "Gasflasche"=10000, "Gasflaschen Nr.:"="", "Ablaufdatum"=timestamp(0 s since 1904-01-01), "Modus"=0, "Komponenten"={"Komponente 1"={"Komponente:"=0, "Konzentration IST"=0.0, "Einheit"=enum."ppm", "Genauigkeit"=0.0}, "Komponente 2"={"Komponente:"=0, "Konzentration IST"=0.0, "Einheit"=enum."ppm", "Genauigkeit"=0.0}, "Komponente 3"={"Komponente:"=0, "Konzentration IST"=0.0, "Einheit"=enum."ppm", "Genauigkeit"=0.0}, "Komponente 4"={"Komponente:"=0, "Konzentration IST"=0.0, "Einheit"=enum."ppm", "Genauigkeit"=0.0}, "Komponente 5"={"Komponente:"=0, "Konzentration IST"=0.0, "Einheit"=enum."ppm", "Genauigkeit"=0.0}}}, {"Span Inlet Active"=FALSE, "Analysator"="", "Konfig Gasflasche"=FALSE, "Gasflasche"=10000, "Gasflaschen Nr.:"="", "Ablaufdatum"=timestamp(0 s since 1904-01-01), "Modus"=0, "Komponenten"={"Komponente 1"={"Komponente:"=0, "Konzentration IST"=0.0, "Einheit"=enum."ppm", "Genauigkeit"=0.0}, "Komponente 2"={"Komponente:"=0, "Konzentration IST"=0.0, "Einheit"=enum."ppm", "Genauigkeit"=0.0}, "Komponente 3"={"Komponente:"=0, "Konzentration IST"=0.0, "Einheit"=enum."ppm", "Genauigkeit"=0.0}, "Komponente 4"={"Komponente:"=0, "Konzentration IST"=0.0, "Einheit"=enum."ppm", "Genauigkeit"=0.0}, "Komponente 5"={"Komponente:"=0, "Konzentration IST"=0.0, "Einheit"=enum."ppm", "Genauigkeit"=0.0}}}, {"Span Inlet Active"=FALSE, "Analysator"="", "Konfig Gasflasche"=FALSE, "Gasflasche"=10000, "Gasflaschen Nr.:"="", "Ablaufdatum"=timestamp(0 s since 1904-01-01), "Modus"=0, "Komponenten"={"Komponente 1"={"Komponente:"=0, "Konzentration IST"=0.0, "Einheit"=enum."ppm", "Genauigkeit"=0.0}, "Komponente 2"={"Komponente:"=0, "Konzentration IST"=0.0, "Einheit"=enum."ppm", "Genauigkeit"=0.0}, "Komponente 3"={"Komponente:"=0, "Konzentration IST"=0.0, "Einheit"=enum."ppm", "Genauigkeit"=0.0}, "Komponente 4"={"Komponente:"=0, "Konzentration IST"=0.0, "Einheit"=enum."ppm", "Genauigkeit"=0.0}, "Komponente 5"={"Komponente:"=0, "Konzentration IST"=0.0, "Einheit"=enum."ppm", "Genauigkeit"=0.0}}}, {"Span Inlet Active"=FALSE, "Analysator"="", "Konfig Gasflasche"=FALSE, "Gasflasche"=10000, "Gasflaschen Nr.:"="", "Ablaufdatum"=timestamp(0 s since 1904-01-01), "Modus"=0, "Komponenten"={"Komponente 1"={"Komponente:"=0, "Konzentration IST"=0.0, "Einheit"=enum."ppm", "Genauigkeit"=0.0}, "Komponente 2"={"Komponente:"=0, "Konzentration IST"=0.0, "Einheit"=enum."ppm", "Genauigkeit"=0.0}, "Komponente 3"={"Komponente:"=0, "Konzentration IST"=0.0, "Einheit"=enum."ppm", "Genauigkeit"=0.0}, "Komponente 4"={"Komponente:"=0, "Konzentration IST"=0.0, "Einheit"=enum."ppm", "Genauigkeit"=0.0}, "Komponente 5"={"Komponente:"=0, "Konzentration IST"=0.0, "Einheit"=enum."ppm", "Genauigkeit"=0.0}}}, {"Span Inlet Active"=FALSE, "Analysator"="", "Konfig Gasflasche"=FALSE, "Gasflasche"=10000, "Gasflaschen Nr.:"="", "Ablaufdatum"=timestamp(0 s since 1904-01-01), "Modus"=0, "Komponenten"={"Komponente 1"={"Komponente:"=0, "Konzentration IST"=0.0, "Einheit"=enum."ppm", "Genauigkeit"=0.0}, "Komponente 2"={"Komponente:"=0, "Konzentration IST"=0.0, "Einheit"=enum."ppm", "Genauigkeit"=0.0}, "Komponente 3"={"Komponente:"=0, "Konzentration IST"=0.0, "Einheit"=enum."ppm", "Genauigkeit"=0.0}, "Komponente 4"={"Komponente:"=0, "Konzentration IST"=0.0, "Einheit"=enum."ppm", "Genauigkeit"=0.0}, "Komponente 5"={"Komponente:"=0, "Konzentration IST"=0.0, "Einheit"=enum."ppm", "Genauigkeit"=0.0}}}, {"Span Inlet Active"=FALSE, "Analysator"="", "Konfig Gasflasche"=FALSE, "Gasflasche"=10000, "Gasflaschen Nr.:"="", "Ablaufdatum"=timestamp(0 s since 1904-01-01), "Modus"=0, "Komponenten"={"Komponente 1"={"Komponente:"=0, "Konzentration IST"=0.0, "Einheit"=enum."ppm", "Genauigkeit"=0.0}, "Komponente 2"={"Komponente:"=0, "Konzentration IST"=0.0, "Einheit"=enum."ppm", "Genauigkeit"=0.0}, "Komponente 3"={"Komponente:"=0, "Konzentration IST"=0.0, "Einheit"=enum."ppm", "Genauigkeit"=0.0}, "Komponente 4"={"Komponente:"=0, "Konzentration IST"=0.0, "Einheit"=enum."ppm", "Genauigkeit"=0.0}, "Komponente 5"={"Komponente:"=0, "Konzentration IST"=0.0, "Einheit"=enum."ppm", "Genauigkeit"=0.0}}}] ("Spangaseinstellungen"), s=w84, f=w82) -> (s? t:f=w81:T2[])
        n36 = call <vilib>:"Clear Errors.vi"("error in (no error)"=w101) -> ()  [unwired: 5 in, 2 out]
      }
      frame "speichern" {
        n37 = Bundle("Drift Konfig Daten"=w135, "Spangaseinstellungen"=w134) -> (w133:T13)  [unwired: 1 in]
        n38 = call "Datei im Ordner des VI (EXE).vi"("Dateiname"="Drift Test Config.bin") -> ("Dateipfad im Ordner des Haupt-VIs"=w143:path)  [unwired: 8 in, 2 out]
        n39 = Open/Create/Replace File(file path (use dialog)=w143, operation (0:open)=T12."open or create" ("Operation (0:open)")) -> (refnum out=w142:refnum<file>, error out=w144:errorcluster)  [unwired: 4 in, 1 out]
        n40 = Write to Binary File(file (use dialog)=w142, data=w133, error in=w144) -> (refnum out=w141:refnum<file>, error out=w140:errorcluster)  [unwired: 3 in, 1 out]
        n41 = Close File(refnum=w141, error in=w140) -> (error out=w139:errorcluster)  [unwired: 1 out]
        n42 = call <vilib>:"Clear Errors.vi"("error in (no error)"=w139) -> ()  [unwired: 5 in, 2 out]
      }
      frame "Tabelle init" {
        n43 = Initialize Array("", 100 ("Dimensionsgröße"), 20 ("Dimensionsgröße")) -> (w153:string[][])
      }
      frame "Tabelle löschen" {
        n44 = Initialize Array("", 100 ("Dimensionsgröße"), 20 ("Dimensionsgröße")) -> (w163:string[][])
      }
      frame "Zeile Prüfen" {
        # "die ersten 4 spalten in der Zeile nicht gefüllt"
        n45 = Index Array(array=w176) -> (element=w177:string[])  [unwired: 2 in]
        n46 = for {
          N: 6 -> [_]
          tunnel: w177 -> [w181] mode=indexing
          tunnel: [w179] -> w173 mode=indexing
          n47 = Equal?(x=w181, y="") -> (x = y?=w179:bool)
        }
        n48 = Boolean Array To Number(Boolean array=w173) -> (number=w174:u32)
        "Zahl" <- w174
        n49 = Greater Or Equal?(x=w174, y=u32 31) -> (x >= y?=→"keine Pre Daten vorhanden":bool)
      }
      frame "Info schreiben" {
        n50 = Index Array(array=w192, index=w186) -> (element=w190:i32)
        n51 = Decrement(x=w190) -> (x-1=w184:i32)
        n52 = call "Info schreiben.vi"("Spaninlet"=w184, "Spangaseinstellungen"=w191) -> ("Array"=w187:T14[][])  [unwired: 12 in, 1 out]
        n53 = Index Array(array=w185, index=w186) -> (element=w183:i32)
        n54 = call "2D in 2D ersetzen.vi"("Teilarray"=w187, "Zeile"=w183, "Eingangs Array"=w189) -> ("Ausgangs Array"=w188:string[][])  [unwired: 7 in, 1 out]
      }
      frame "Span Einstellung" {
        n55 = property class="RKElem"(reference=w198) -> (error out=w196:errorcluster, "Pages"=w197:refnum<vi>[])  [unwired: 1 in, 1 out]
        n56 = call <vilib>:"Clear Errors.vi"("error in (no error)"=w196) -> ()  [unwired: 5 in, 2 out]
        n57 = for {
          tunnel: "Spangaseinstellungen" -> [w211] mode=indexing
          tunnel: w197 -> [w204] mode=indexing
          n58 = Unbundle By Name(w211) -> ("Span Inlet Active"=w205:T3)
          n59 = Select(t=u32 6618880, s=w205, f=u32 15066597) -> (s? t:f=w209:u32)
          n60 = property class="Seite"(reference=w204, "FG Color"=w209, "BG Color"=u32 16777226) -> (error out=w210:errorcluster)  [unwired: 1 in, 1 out]
          n61 = call <vilib>:"Clear Errors.vi"("error in (no error)"=w210) -> ()  [unwired: 5 in, 2 out]
        }
        n62 = call "Tabellen Index Manager.vi"("Spangaseinstellungen"="Spangaseinstellungen") -> ("Tabellenbeginn"=w200:i32[], "Verwendete Spangaseingänge"=w199:i32[])  [unwired: 12 in, 1 out]
      }
      frame "Pre Werte schreiben" {
        n63 = Index Array(array=w225, index=w223) -> (element=w224:i32)
        n64 = Index Array(array=w222, index=w223) -> (element=w218:i32)
        n65 = Decrement(x=w224) -> (x-1=w213:i32)
        n66 = call "Driftmessdaten sammeln.vi"("Spaninlet"=w213, "Spangaseinstellungen"=w226) -> ("Messdaten"=w229:sgl[])  [unwired: 12 in, 1 out]
        n67 = Select(t=6 ("Spalte"), s=w217, f=7 ("Spalte")) -> (s? t:f=w214:i32)
        n68 = Number To Fractional String(number=w229) -> (F-format string=w219:string[])  [unwired: 3 in]
        n69 = call "2D Array Teil ersetzen.vi"("Neues Element/Teil-Array"=w219, "Spalte"=w214, "Zeile"=w218, "Eingangs Array"=w221) -> ("Ausgangs Array"=w220:string[][])  [unwired: 7 in]
      }
      frame "NB Pre Wert schreiben" {
        n70 = Index Array(array=w234, index=w235) -> (element=w233:T15)
        n71 = Unbundle By Name(w233) -> ("Tabellenbeginn"=w231:i32, "Spangaseingang"=w232:i32)
        n72 = call "Driftmessdaten sammeln.vi"("Spaninlet"=w232, "Spangaseinstellungen"=w242) -> ("Messdaten"=w245:sgl[])  [unwired: 12 in, 1 out]
        n73 = Number To Fractional String(number=w245) -> (F-format string=w237:string[])  [unwired: 3 in]
        n74 = call "2D Array Teil ersetzen.vi"("Neues Element/Teil-Array"=w237, "Spalte"=7, "Zeile"=w231, "Eingangs Array"=w239) -> ("Ausgangs Array"=w238:string[][])  [unwired: 7 in]
      }
      frame "NB Post Wert schreiben" {
        n75 = Index Array(array=w250, index=w251) -> (element=w249:T15)
        n76 = Unbundle By Name(w249) -> ("Tabellenbeginn"=w247:i32, "Spangaseingang"=w248:i32)
        n77 = call "Driftmessdaten sammeln.vi"("Spaninlet"=w248, "Spangaseinstellungen"=w258) -> ("Messdaten"=w261:sgl[])  [unwired: 12 in, 1 out]
        n78 = Number To Fractional String(number=w261) -> (F-format string=w253:string[])  [unwired: 3 in]
        n79 = call "2D Array Teil ersetzen.vi"("Neues Element/Teil-Array"=w253, "Spalte"=9, "Zeile"=w247, "Eingangs Array"=w255) -> ("Ausgangs Array"=w254:string[][])  [unwired: 7 in]
      }
      frame "Post Werte schreiben" {
        n80 = Index Array(array=w273, index=w274) -> (element=w269:i32)
        n81 = Index Array(array=w275, index=w274) -> (element=w264:i32)
        n82 = Decrement(x=w264) -> (x-1=w263:i32)
        n83 = call "Driftmessdaten sammeln.vi"("Spaninlet"=w263, "Spangaseinstellungen"=w276) -> ("Messdaten"=w279:sgl[])  [unwired: 12 in, 1 out]
        n84 = Select(t=8 ("Spalte"), s=w268, f=9 ("Spalte")) -> (s? t:f=w265:i32)
        n85 = Number To Fractional String(number=w279) -> (F-format string=w270:string[])  [unwired: 3 in]
        n86 = call "2D Array Teil ersetzen.vi"("Neues Element/Teil-Array"=w270, "Spalte"=w265, "Zeile"=w269, "Eingangs Array"=w272) -> ("Ausgangs Array"=w271:string[][])  [unwired: 7 in]
      }
    }
  }
  "Drift Konfig Daten" <- w6
  "Drifttabelle" <- w5
  "Spangaseinstellungen" <- w4
  "Verwendete Spangaseingänge" <- w3
  "Tabellenbeginn" <- w2
  "PDF Pfad" <- w1
